vi "Cut Impulse.vi"(0 "Sample Rate":i32, 1 "Impulse Direction +ve?":bool, 2 "Cut region":enum16{"Before", "After"}(ring), 3 "X Position":i32, 4 "Impulse Plane":T2(ring), 5 "Impulse Positions (in)":T1(array[cluster]) {"Amplitude offset" format="%.2f"}) -> (19 "Impulse Positions (out)":T1(array[cluster]) {"Amplitude offset" format="%.2f"})   [LabVIEW 2013, in "impulse functions.lvlib"]
uses:
  impulse functions.lvlib
panel:
  # "Copyright Americo A. Migliaccio (c) 2002 All Rights Reserved by Author"
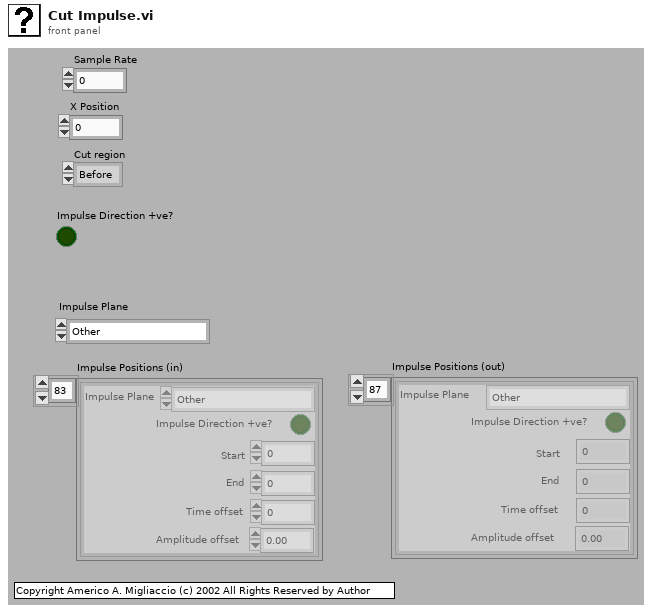
[diagram p1: front panel]
types:
  T1 = cluster{"Start":i32, "End":i32, "Impulse Plane":enum16{"Other", "Yaw", "Pitch", "Roll", "LARP", "RALP"}, "Impulse Direction +ve?":bool, "Time offset":i32, "Amplitude offset":dbl}[]
  T2 = enum16{"Other", "Yaw", "Pitch", "Roll", "LARP", "RALP"}
  T3 = cluster{"Start":i32, "End":i32, "Impulse Plane":enum16{"Other", "Yaw", "Pitch", "Roll", "LARP", "RALP"}, "Impulse Direction +ve?":bool, "Time offset":i32, "Amplitude offset":dbl}
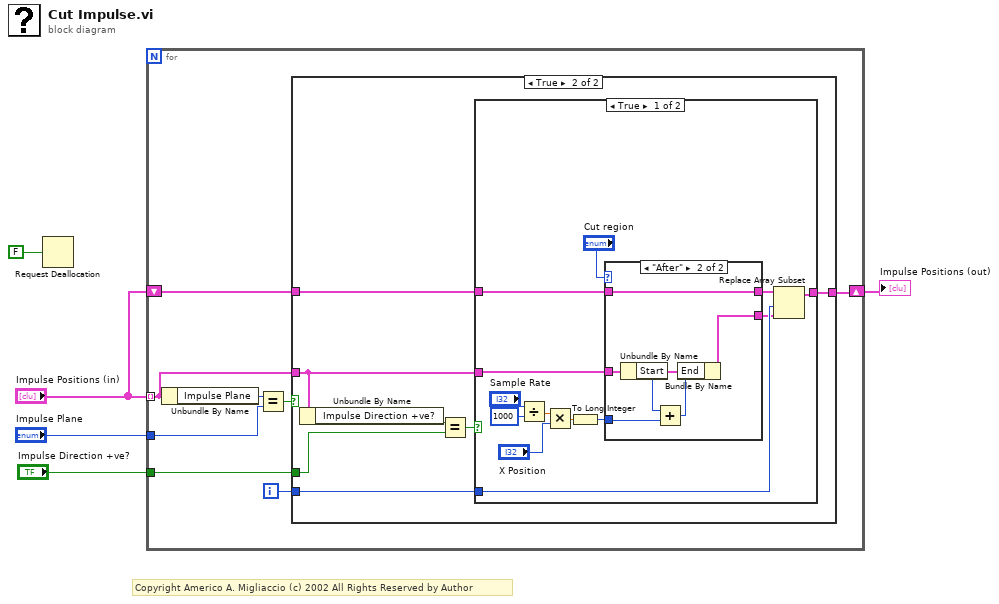
[diagram p0: block diagram]
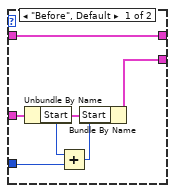
[diagram p3: hidden frame]
diagram:
  # "Copyright Americo A. Migliaccio (c) 2002 All Rights Reserved by Author"
  n1 = Request Deallocation(FALSE ("flag")) -> ()
  n2 = for {
    tunnel: "Impulse Positions (in)" -> [w10] mode=indexing
    tunnel: "Impulse Plane" -> [w12]
    tunnel: "Impulse Direction +ve?" -> [w9]
    shift-right: [w7] -> w2
    shift-left: "Impulse Positions (in)" -> [w8]
    i -> [w6]
    n3 = Unbundle By Name(w10) -> ("Impulse Plane"=w13:T2)
    n4 = Equal?(x=w13, y=w12) -> (x = y?=w11:bool)
    n5 = case shown="True" w11 {
      tunnel: w10 -> [_ w21]
      tunnel: w9 -> [_ w20]
      tunnel: w8 -> [w14 w17]
      tunnel: [w14 w15] -> w7
      tunnel: w6 -> [_ w16]
      frame False {
      }
      frame True {
        n6 = Unbundle By Name(w21) -> ("Impulse Direction +ve?"=w18:bool)
        n7 = Equal?(x=w18, y=w20) -> (x = y?=w19:bool)
        n8 = case shown="True" w19 {
          tunnel: w21 -> [w28 _]
          tunnel: w17 -> [w34 w47]
          tunnel: [w32 w47] -> w15
          tunnel: w16 -> [w31 _]
          frame True {
            n9 = Divide(x="Sample Rate", y=1000) -> (x/y=w24:dbl)
            n10 = Multiply(x=w24, y="X Position") -> (x*y=w22:dbl)
            n11 = To Long Integer(number=w22) -> (32bit integer=w23:i32)
            n12 = case shown="\"After\"" "Cut region" {
              tunnel: w34 -> [w39 w45]
              tunnel: [w39 w45] -> w33
              tunnel: [w38 w44] -> w30
              tunnel: w28 -> [w40 w46]
              tunnel: w23 -> [w37 w43]
              frame "Before", Default {
                n13 = Unbundle By Name(w40) -> ("Start"=w36:i32)
                n14 = Add(x=w36, y=w37) -> (x+y=w35:i32)
                n15 = Bundle By Name(cluster=w40, "Start"=w35) -> (w38:T3)
              }
              frame "After" {
                n16 = Unbundle By Name(w46) -> ("Start"=w42:i32)
                n17 = Add(x=w42, y=w43) -> (x+y=w41:i32)
                n18 = Bundle By Name(cluster=w46, "End"=w41) -> (w44:T3)
              }
            }
            n19 = Replace Array Subset(array=w33, new element=w30, index=w31) -> (w32:T1)
          }
          frame False {
          }
        }
      }
    }
  }
  "Impulse Positions (out)" <- w2
